vi "stop_subsystem_pv.vi"(9 "port":u16, 10 "host":string, 11 "path in":path=path "hl2ss_ulm.dll") -> (0 "error":bool, 1 "port":u16, 2 "host":string, 3 "path out":path)   [LabVIEW 2023]
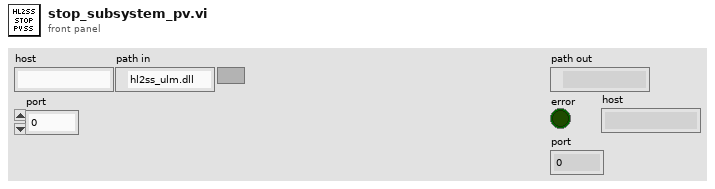
[diagram p1: front panel]
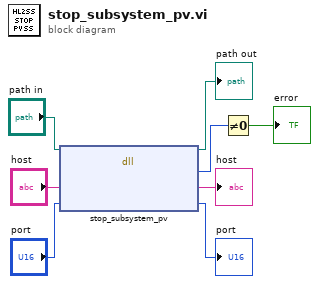
[diagram p0: block diagram]
diagram:
  n1 = dll-call lib="C:/Users/jcds/Documents/GitHub/hl2ss/extensions/client_labview/hl2ss_ulm.dll" fn="stop_subsystem_pv"(path in="path in", "host"="host", "port"="port") -> (path out=→"path out":path, "return type"=w4:i32, "host"=→"host":string, "port"=→"port":u16)  [unwired: 2 in, 1 out]
  n2 = Not Equal To 0?(x=w4) -> (x != 0?=→"error":bool)
